vi "query.vi"(3 "error in (no error)":errorcluster, 4 "string_in":string, 5 "VISA in":refnum<visa-resource-name>="COM5") -> (0 "error out":errorcluster, 1 "read buffer":string, 2 "VISA out":refnum<visa-resource-name>)   [LabVIEW 2020]
panel:
  in  "stop":bool
  out "Number of Bytes at Port":u32
  out "return count":u32
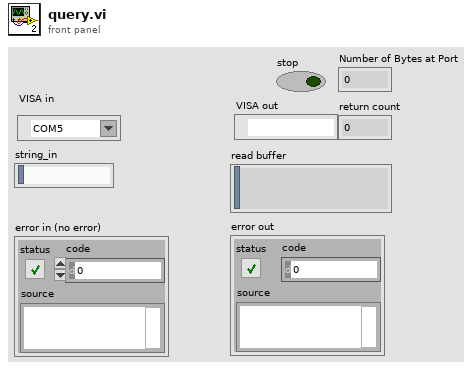
[diagram p1: front panel]
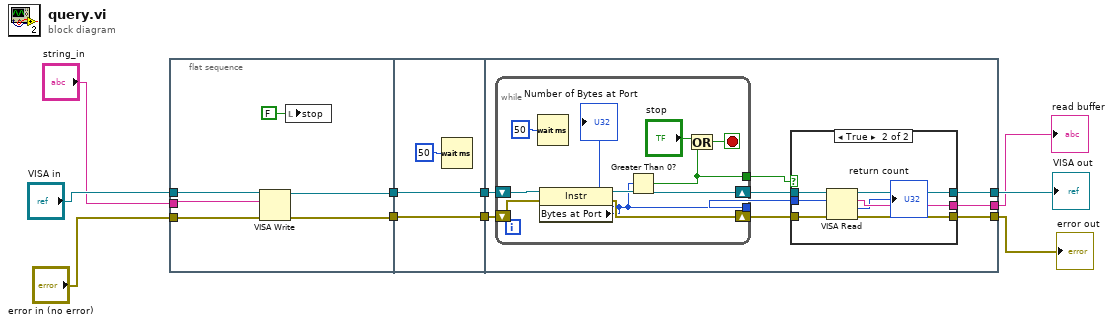
[diagram p0: block diagram]
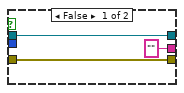
[diagram p2: hidden frame]
diagram:
  n1 = flat-sequence {
    tunnel: [w16] -> w10
    tunnel: [w15] -> w9
    tunnel: "error in (no error)" -> [w14]
    tunnel: "string_in" -> [w13]
    tunnel: "VISA in" -> [w12]
    tunnel: w10 -> [w19]
    tunnel: [w19] -> w8
    tunnel: w9 -> [w18]
    tunnel: [w18] -> w7
    tunnel: w8 -> [w25]
    tunnel: w7 -> [w24]
    tunnel: [w28] -> w6
    tunnel: [w26] -> w3
    tunnel: [w27] -> w2
    frame #0 {
      n2 = VISA Write(VISA resource name=w12, write buffer=w13, error in (no error)=w14) -> (VISA resource name out=w16:refnum<visa-resource-name>, error out=w15:errorcluster)  [unwired: 1 out]
      n3 = local write "stop"(FALSE ("stop")) -> ()
    }
    frame #1 {
      n4 = Wait (ms)(milliseconds to wait=u32 50) -> ()  [unwired: 1 out]
    }
    frame #2 {
      n5 = while {
        tunnel: [w43] -> w21
        shift-right: [w45] -> w23
        shift-left: w25 -> [w47]
        shift-right: [w44] -> w22
        shift-left: w24 -> [w46]
        tunnel: [w39] -> w20
        stop <- w42 stop-if-true
        n6 = Wait (ms)(milliseconds to wait=u32 50) -> ()  [unwired: 1 out]
        n7 = property class="Instr"(reference=w47, error in=w46) -> (reference out=w45:refnum<visa-resource-name>, error out=w44:errorcluster, "Bytes at Port"=w43:u32)
        "Number of Bytes at Port" <- w43
        n8 = Greater Than 0?(x=w43) -> (x > 0?=w39:bool)
        n9 = Or(x="stop", y=w39) -> (x .or. y?=w42:bool)
      }
      n10 = case shown="True" w20 {
        tunnel: [w31 w38] -> w28
        tunnel: ["" ("read buffer") w37] -> w27
        tunnel: [w30 w36] -> w26
        tunnel: w23 -> [w31 w35]
        tunnel: w22 -> [w30 w34]
        tunnel: w21 -> [_ w33]
        frame False {
        }
        frame True {
          n11 = VISA Read(VISA resource name=w35, byte count=w33, error in (no error)=w34) -> (VISA resource name out=w38:refnum<visa-resource-name>, read buffer=w37:string, return count=→"return count":u32, error out=w36:errorcluster)
        }
      }
    }
  }
  "error out" <- w3
  "read buffer" <- w2
  "VISA out" <- w6
